vi "CalcCubeDuration.vi"(8 "error in (no error)":errorcluster, 11 "Acquisition in":refnum<class "Acquisition.lvclass">) -> (0 "error out":errorcluster, 3 "Acquisition out":refnum<class "Acquisition.lvclass">)   [LabVIEW 2018, in "Acquisition.lvclass"]
uses:
  Acquisition.lvclass
  Acquisition.lvclass/Acquisition.ctl
  Interface/Interface.lvclass/Interface.ctl
  Channel/Channel.lvclass
  Interface/Interface.lvclass
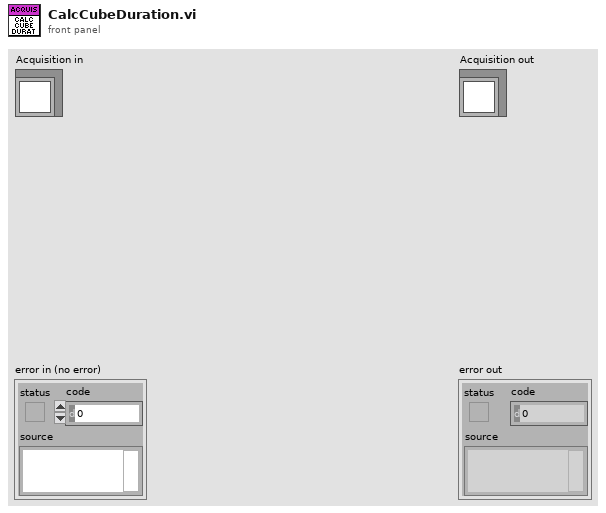
[diagram p1: front panel]
types:
  T1 = cluster{"ACQUISITION_MODE":u8, "TRIGGER_MODE":u8, "READ_MODE":u8, "PREAMP":u8, "READOUT_RATE":u8, "VERTICAL_SHIFT_SPEED":u8, "EM_MODE":u8, "EM_GAIN":u16, "SHUTTER_MODE":u8, "SHUTTER_TTL":u8, "SHUTTER_OPENING_TIME":u16, "SHUTTER_CLOSING_TIME":u16, "VBIN":u16, "HBIN":u16, "INITIAL_LINE":u16, "INITIAL_COLUMN":u16, "FINAL_LINE":u16, "FINAL_COLUMN":u16, "FRAME_TRANSFER":bool, "VERTICAL_CLOCK_VOLTAGE":u8, "AD_CHANNEL":u32}
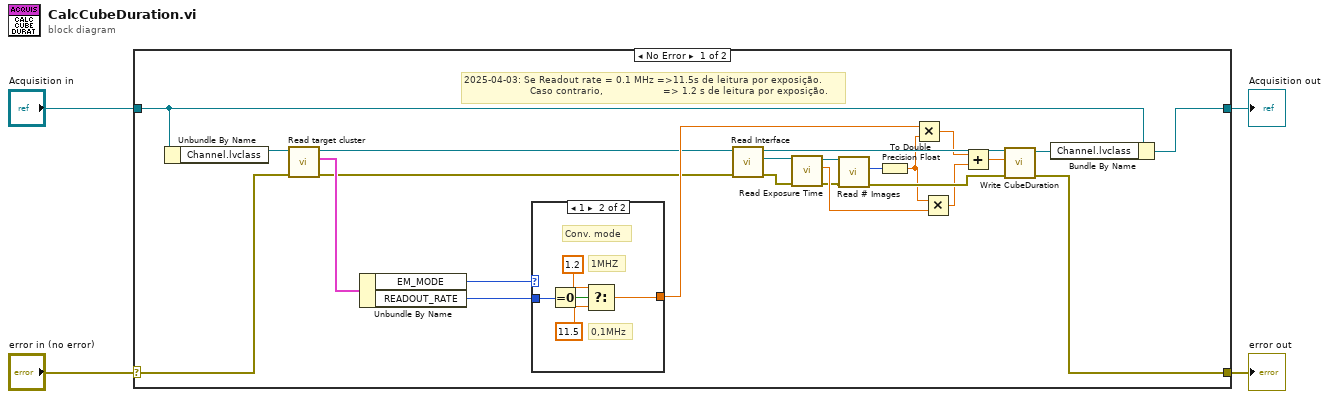
[diagram p0: block diagram]
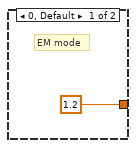
[diagram p2: hidden frame]
diagram:
  n1 = case shown="No Error" "error in (no error)" {
    selector: "error in (no error)" -> [w11 w36]
    tunnel: [w17 w36] -> w3
    tunnel: [w21 w35] -> w1
    tunnel: "Acquisition in" -> [w23 w35]
    frame No Error {
      # "2025-04-03: Se Readout rate = 0.1 MHz =>11.5s de leitura por exposição.\n                      Caso contrario,                    => 1.2 s de leitura por exposição."
      n2 = Unbundle By Name(w23) -> ("Channel.lvclass"=w12:refnum<class "Channel.lvclass">)
      n3 = call-dynamic "Read target cluster.vi"("error in (no error)"=w11, "Channel in"=w12) -> ("error out"=w6:errorcluster, "target cluster"=w10:T1, "Channel out"=w5:refnum<class "Channel.lvclass">)  [unwired: 7 in]
      n4 = Unbundle By Name(w10) -> ("EM_MODE"=w9:u8, "READOUT_RATE"=w8:u8)
      n5 = case shown="1" w9 {
        tunnel: [1.2 ("x") w30] -> w7
        tunnel: w8 -> [_ w34]
        frame 0, Default {
          # "EM mode"
        }
        frame 1 {
          # "0,1MHz"
          # "1MHZ"
          # "Conv. mode"
          n6 = Equal To 0?(x=w34) -> (x = 0?=w33:bool)
          n7 = Select(t=1.2 ("x"), s=w33, f=11.5) -> (s? t:f=w30:dbl)
        }
      }
      n8 = call-dynamic "Read Interface.vi"("error in (no error)"=w6, "Channel in"=w5) -> ("error out"=w20:errorcluster, "Interface.lvclass"=w26:refnum<class "Interface.lvclass">, "Channel out"=w24:refnum<class "Channel.lvclass">)  [unwired: 7 in]
      n9 = call "Read Exposure Time.vi"("error in (no error)"=w20, "Interface in"=w26) -> ("error out"=w19:errorcluster, "Exposure Time"=w27:dbl, "Interface out"=w25:refnum<class "Interface.lvclass">)  [unwired: 7 in]
      n10 = call-dynamic "Read # Images.vi"("error in (no error)"=w19, "Interface in"=w25) -> ("error out"=w18:errorcluster, "# Images"=w28:u32)  [unwired: 7 in, 1 out]
      n11 = To Double Precision Float(number=w28) -> (double precision float=w13:dbl)
      n12 = Multiply(x=w7, y=w13) -> (x*y=w14:dbl)
      n13 = Multiply(x=w13, y=w27) -> (x*y=w15:dbl)
      n14 = Add(x=w14, y=w15) -> (x+y=w16:dbl)
      n15 = call-dynamic "Write CubeDuration.vi"("error in (no error)"=w18, "CubeDuration"=w16, "Channel in"=w24) -> ("error out"=w17:errorcluster, "Channel out"=w22:refnum<class "Channel.lvclass">)  [unwired: 7 in]
      n16 = Bundle By Name(cluster=w23, "Channel.lvclass"=w22) -> (w21:refnum<class "Acquisition.lvclass">)
    }
    frame Error {
    }
  }
  "error out" <- w3
  "Acquisition out" <- w1
